vi "Test Re-entrancy.vi"(10 "Folder Path":path) -> (2 "All Re-entrant?":bool)   [LabVIEW 2014]
panel:
  out "Array":bool[](array[boolean])
  out "Iteration":i32
  out "All Files in Dir":path[](array[path])
  out "Total Number of Files?":i32
  out "File Failed?":path
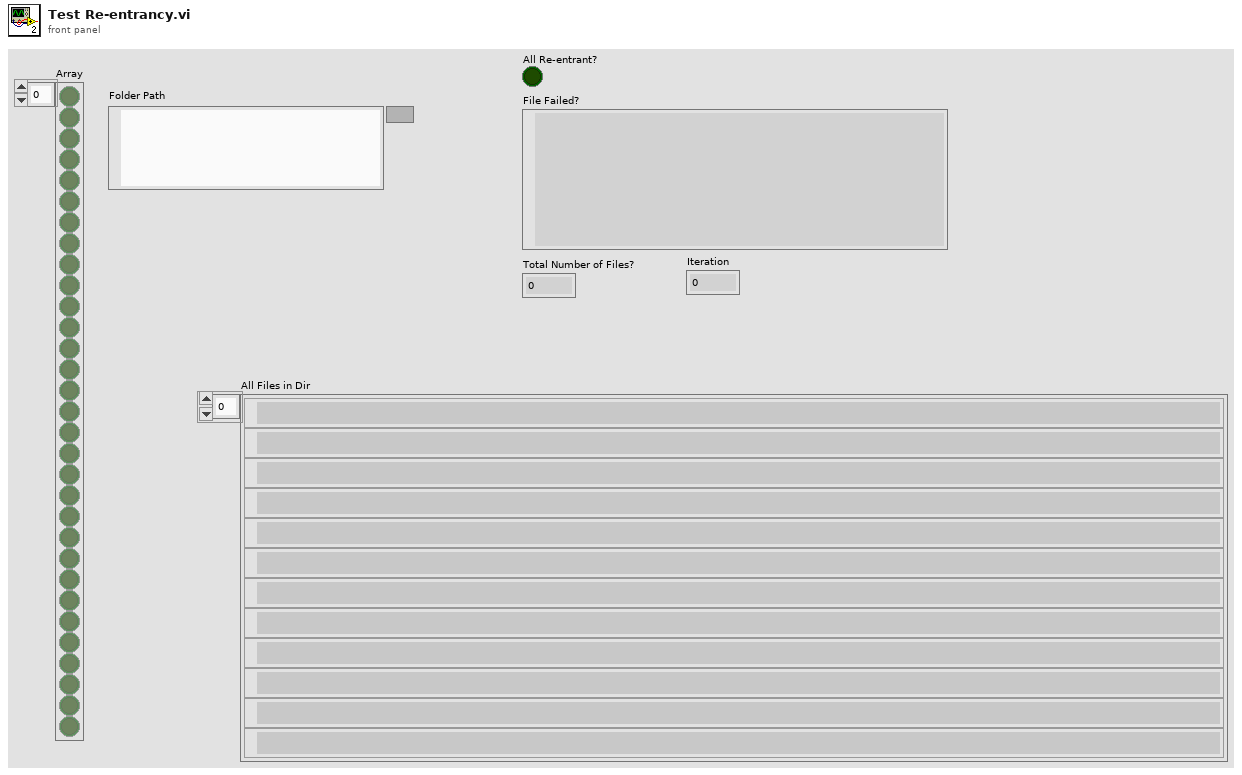
[diagram p1: front panel]
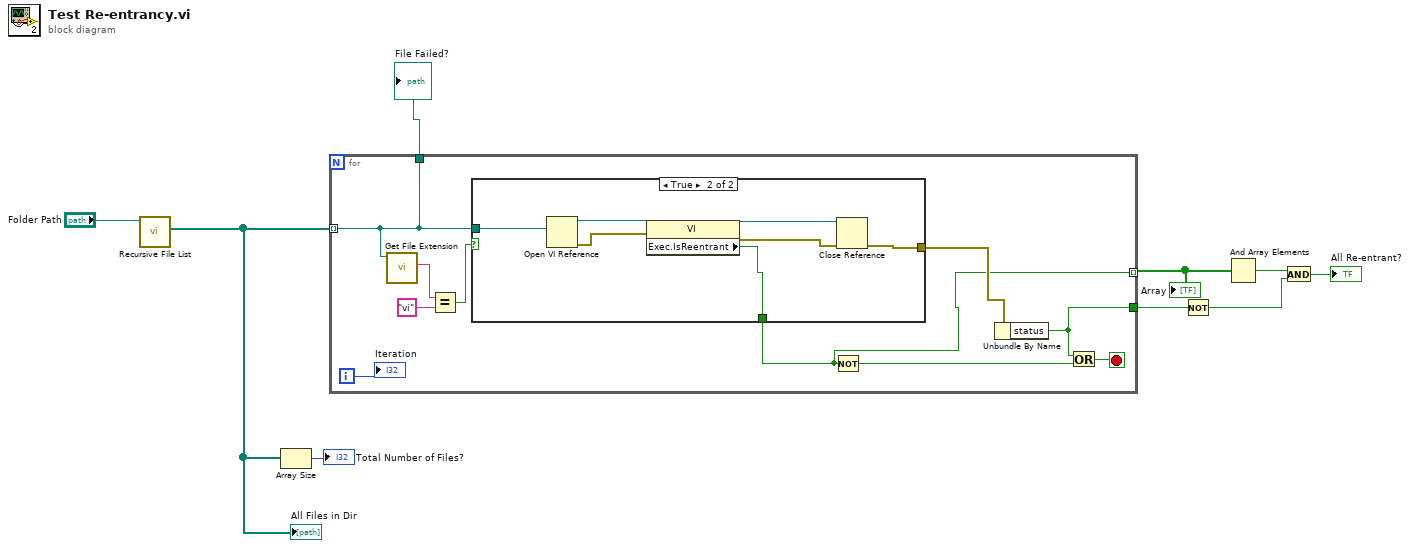
[diagram p0: block diagram]
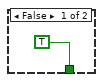
[diagram p2: hidden frame]
diagram:
  n1 = call <vilib>:"Recursive File List.vi"("Folder Path"="Folder Path") -> ("All Files in Dir"=w4:path[])  [unwired: 6 in, 4 out]
  "All Files in Dir" <- w4
  n2 = Array Size(array=w4) -> (size(s)=→"Total Number of Files?":i32)
  n3 = for {
    tunnel: w4 -> [w16] mode=indexing
    tunnel: [w11] -> w8 mode=indexing
    tunnel: [w16] -> w5
    tunnel: [w10] -> w2
    i -> [w15]
    stop <- w14 stop-if-true
    n4 = call <vilib>:"Get File Extension.vi"("file"=w16) -> ("lowercase file extension"=w19:string)  [unwired: 7 in, 3 out]
    n5 = Equal?(x=w19, y="vi") -> (x = y?=w17:bool)
    n6 = case shown="True" w17 {
      tunnel: [_ w23] -> w13
      tunnel: w16 -> [_ w22]
      tunnel: [TRUE ("Exec.IsReentrant") w21] -> w11
      frame False {
      }
      frame True {
        n7 = Open VI Reference(vi path=w22) -> (vi reference=w27:refnum<vi>, error out=w26:errorcluster)  [unwired: 5 in]
        n8 = property class="VI"(reference=w27, error in=w26) -> (reference out=w25:refnum<vi>, error out=w24:errorcluster, "Exec.IsReentrant"=w21:bool)
        n9 = Close Reference(reference=w25, error in (no error)=w24) -> (error out=w23:errorcluster)
      }
    }
    n10 = Not(x=w11) -> (.not. x?=w12:bool)
    n11 = Unbundle By Name(w13) -> ("status"=w10:bool)
    n12 = Or(x=w10, y=w12) -> (x .or. y?=w14:bool)
    "Iteration" <- w15
  }
  "File Failed?" <- w5
  "Array" <- w8
  n13 = Not(x=w2) -> (.not. x?=w1:bool)
  n14 = And Array Elements(Boolean array=w8) -> (logical AND=w7:bool)
  n15 = And(x=w7, y=w1) -> (x .and. y?=→"All Re-entrant?":bool)
